vi "Set Producer Values.vi"(8 "error in":errorcluster, 9 "Producer Ch":T2[](array[typedef])=[{"Error.STS"=0, "OutputEnable.STS"=0, "ControlMode.STS"=0, "Voltage.AV"=0.0, "Current.AV"=0.0, "Power.AV"=0.0, "VoltageNominal.AV"=0.0, "CurrentNominal.AV"=0.0, "PowerNominal.AV"=0.0, "ParameterSet.STS"=0}], 10 "Producer Control":T1, 11 "Cycler Cluster.lvclass in":refnum<class "Cycler Cluster.lvclass">) -> (0 "error out":errorcluster, 3 "Cycler Cluster.lvclass out":refnum<class "Cycler Cluster.lvclass">)   [LabVIEW 2023, in "Cycler Cluster.lvclass"]
uses:
  Cycler Cluster.lvclass
  Producer Ch.ctl
  Producer Control.ctl
  Cycler Cluster.lvclass/Cycler Cluster.ctl
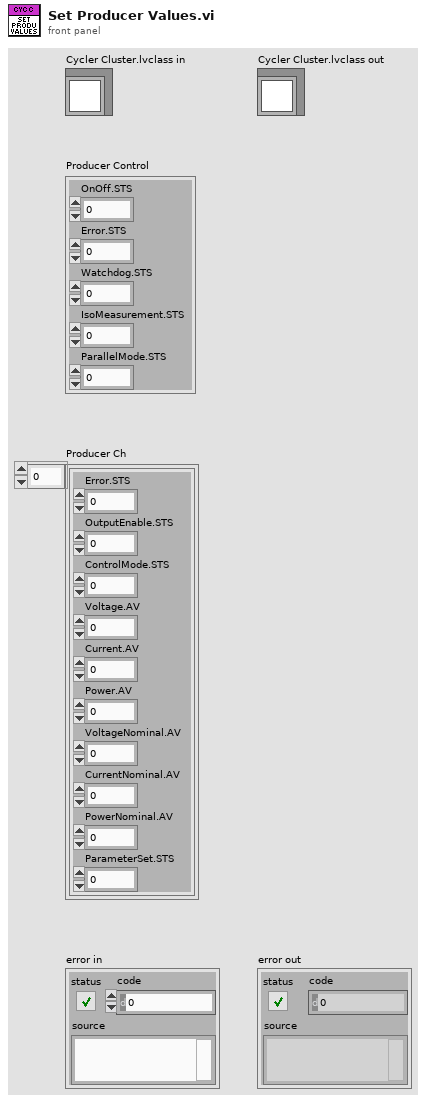
[diagram p1: front panel]
types:
  T1 = typedef "Cycler Cluster.lvclass/Producer Control.ctl" = cluster{"OnOff.STS":i32, "Error.STS":i32, "Watchdog.STS":i32, "IsoMeasurement.STS":i32, "ParallelMode.STS":i32}
  T2 = typedef "Cycler Cluster.lvclass/Producer Ch.ctl" = cluster{"Error.STS":i32, "OutputEnable.STS":i32, "ControlMode.STS":u16, "Voltage.AV":dbl, "Current.AV":dbl, "Power.AV":dbl, "VoltageNominal.AV":dbl, "CurrentNominal.AV":dbl, "PowerNominal.AV":dbl, "ParameterSet.STS":i32}
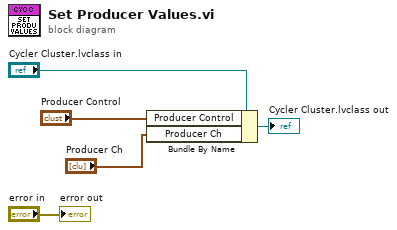
[diagram p0: block diagram]
diagram:
  n1 = Bundle By Name(cluster="Cycler Cluster.lvclass in", "Producer Control"="Producer Control", "Producer Ch"="Producer Ch") -> (→"Cycler Cluster.lvclass out":refnum<class "Cycler Cluster.lvclass">)
  "error out" <- "error in"
